vi "Get Specific Filter Configuration String.vi"(11 "Time Filters in":refnum<class "Time Filters.lvclass">) -> (2 "Filter String":string)   [LabVIEW 2016, in "Assert API Components.lvlib" / "Time Filters.lvclass"]
uses:
  Time Filters.lvclass
  Time Filters.lvclass/Time Filters.ctl
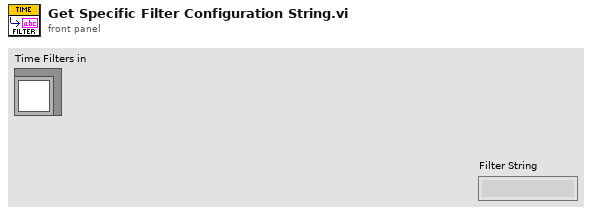
[diagram p1: front panel]
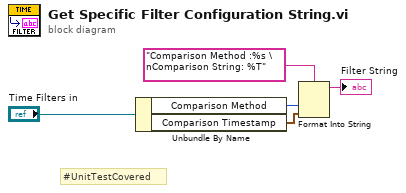
[diagram p0: block diagram]
diagram:
  # "#UnitTestCovered"
  n1 = Unbundle By Name("Time Filters in") -> ("Comparison Method"=w3:enum16{"Before", "After"}, "Comparison Timestamp"=w2:timestamp)
  n2 = Format Into String(format string="Comparison Method :%s \nComparison String: %T", w3, w2) -> (resulting string=→"Filter String":string)  [unwired: 2 in, 1 out]
